vi "LaunchClientUI.vi"   [LabVIEW 2018, in "ClientUI.lvlib"]
uses:
  ClientUI.lvlib
  ClientUI/ClientUI.lvclass
  C:/Program Files/National Instruments/LabVIEW 2018/vi.lib/ActorFramework/Actor/Actor.lvclass
  <vilib>/ActorFramework/Actor/Actor.lvclass
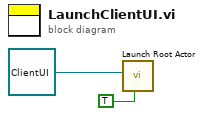
[diagram p0: block diagram]
diagram:
  n1 = call <vilib>:"Launch Root Actor.vi"("Open Actor Core front panel? (F)"=TRUE, "Actor"=refnum<class "ClientUI.lvclass"> refnum ("ClientUI.lvlib:ClientUI.lvclass")) -> ()  [unwired: 8 in, 2 out]
